vi "PWM_in.vi"() -> ()   [LabVIEW 2012]
uses:
  Usb_Daq_V52_Dll.dll
panel:
  in  "通道":i32=1 min=0 max=3
  in  "stop":bool
  in  "read":bool
  out "占空比":sgl
  out "频率":dbl
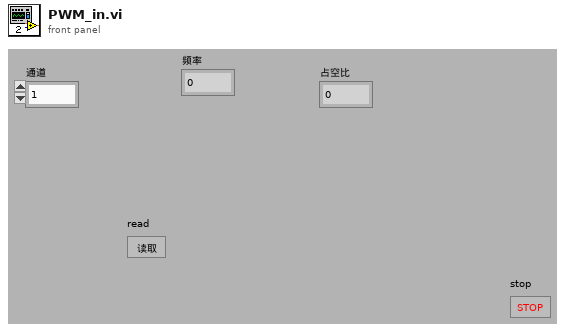
[diagram p1: front panel]
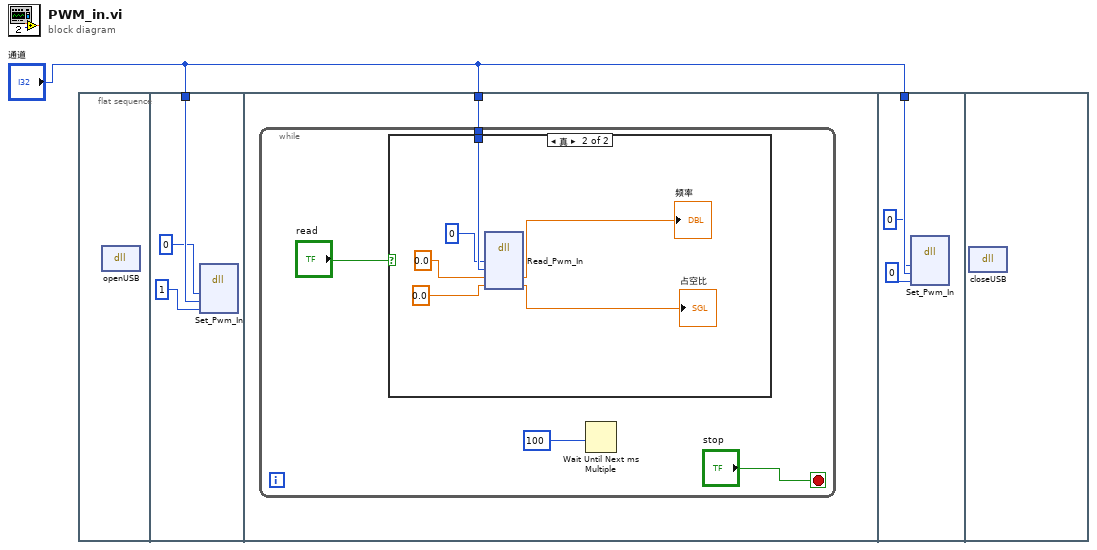
[diagram p0: block diagram]
diagram:
  n1 = flat-sequence {
    tunnel: "通道" -> [w4]
    tunnel: "通道" -> [w5]
    tunnel: "通道" -> [w17]
    frame #0 {
      n2 = dll-call lib="PTH1labs Ebackup数据采集卡uSB!USB数据采集卡资料HKUSB6203例程labviewUsb_Daq_V52_Dll.dll" fn="openUSB"() -> ()  [unwired: 3 in, 3 out]
    }
    frame #1 {
      n3 = dll-call lib="PTH1labs Ebackup数据采集卡uSB!USB数据采集卡资料HKUSB6203例程labviewUsb_Daq_V52_Dll.dll" fn="Set_Pwm_In"("dev"=0, "ch"=w4, "en"=1) -> ()  [unwired: 5 in, 4 out]
    }
    frame #2 {
      n4 = while {
        tunnel: w5 -> [w6]
        stop <- "stop" stop-if-true
        n5 = case shown="真" "read" {
          tunnel: w6 -> [_ w13]
          frame False {
          }
          frame True {
            n6 = dll-call lib="PTH1labs Ebackup数据采集卡uSB!USB数据采集卡资料HKUSB6203例程labviewUsb_Daq_V52_Dll.dll" fn="Read_Pwm_In"("dev"=0, "ch"=w13, "freq"=sgl 0.0, "DutyCycle"=sgl 0.0) -> ("freq"=→"频率":sgl, "DutyCycle"=→"占空比":sgl)  [unwired: 4 in, 4 out]
          }
        }
        n7 = Wait Until Next ms Multiple(millisecond multiple=100) -> ()  [unwired: 1 out]
      }
    }
    frame #3 {
      n8 = dll-call lib="PTH1labs Ebackup数据采集卡uSB!USB数据采集卡资料HKUSB6203例程labviewUsb_Daq_V52_Dll.dll" fn="Set_Pwm_In"("dev"=0, "ch"=w17, "en"=0) -> ()  [unwired: 5 in, 4 out]
    }
    frame #4 {
      n9 = dll-call lib="PTH1labs Ebackup数据采集卡uSB!USB数据采集卡资料HKUSB6203例程labviewUsb_Daq_V52_Dll.dll" fn="closeUSB"() -> ()  [unwired: 3 in, 3 out]
    }
  }
